vi "Stanford Research SR1 Quick Measurements.vi"() -> ()   [LabVIEW 2014]
doc: "This example shows how to configure a Quick Measurement for a free-run and set up a basic structure for stopping and resuming the Distortion Quick Measurement."
uses:
  Stanford Research SR1.lvlib
panel:
  in  "Pause / Resume":bool
  in  "Stop":bool
  in  "Number Of Steps (0)":i32
  in  "Stop Frequency (10 Hz)":dbl=10.0
  in  "Start Frequency (10 Hz)":dbl=10.0
  in  "Waveform (0: wsSine)":i32(ring) items=["wsSine", "wsLDSine"]
  in  "VISA resource name":refnum<visa-resource-name>
  # "(c) 2014 National Instruments.  ALL RIGHTS RESERVED."
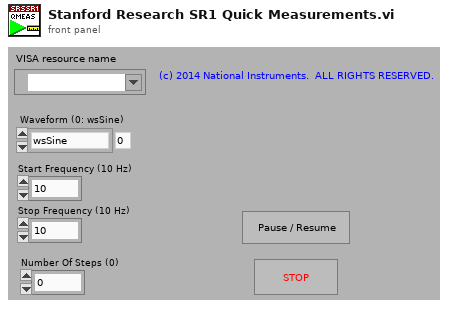
[diagram p1: front panel]
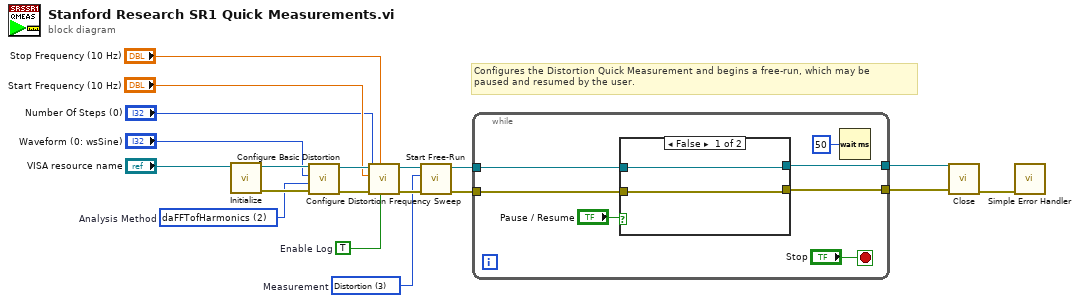
[diagram p0: block diagram]
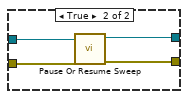
[diagram p2: hidden frame]
diagram:
  w6 = 2 items=["daTHD", "daHarmonics", "daFFTofHarmonics"]  # Analysis Method
  w7 = TRUE  # Enable Log
  w8 = 3 items=["Level", "SNR", "THDN", "Distortion", "IMDistortion", "Crosstalk", "FrequencyResponse", "InputOutputPhase", "InterchannelPhase"]  # Measurement
  # "Configures the Distortion Quick Measurement and begins a free-run, which may be \npaused and resumed by the user."
  n1 = call "Initialize.vi"("VISA resource name"="VISA resource name") -> ("error out"=w16:errorcluster, "VISA resource name out"=w17:refnum<visa-resource-name>)  [unwired: 9 in]
  n2 = call "Configure Basic Distortion.vi"("error in (no error)"=w16, "Analysis Method (0: daTHD)"=w6, "Waveform (0: wsSine)"="Waveform (0: wsSine)", "VISA resource name"=w17) -> ("error out"=w13:errorcluster, "VISA resource name out"=w14:refnum<visa-resource-name>)  [unwired: 6 in]
  n3 = call "Configure Distortion Frequency Sweep.vi"("Enable Log (F: Disabled)"=w7, "Stop Frequency (10 Hz)"="Stop Frequency (10 Hz)", "error in (no error)"=w13, "Number Of Steps (0)"="Number Of Steps (0)", "Start Frequency (10 Hz)"="Start Frequency (10 Hz)", "VISA resource name"=w14) -> ("error out"=w9:errorcluster, "VISA resource name out"=w10:refnum<visa-resource-name>)  [unwired: 4 in]
  n4 = call "Start Free-Run.vi"("error in (no error)"=w9, "Measurement (0: Level)"=w8, "VISA resource name"=w10) -> ("error out"=w3:errorcluster, "VISA resource name out"=w4:refnum<visa-resource-name>)  [unwired: 7 in]
  n5 = while {
    tunnel: w4 -> [w24]
    tunnel: w3 -> [w23]
    tunnel: [w22] -> w2
    tunnel: [w21] -> w1
    stop <- "Stop" stop-if-true
    n6 = case shown="False" "Pause / Resume" {
      tunnel: w24 -> [w28 w32]
      tunnel: w23 -> [w27 w31]
      tunnel: [w28 w30] -> w22
      tunnel: [w27 w29] -> w21
      frame False {
      }
      frame True {
        n7 = call "Pause Or Resume Sweep.vi"("error in (no error)"=w31, "VISA resource name"=w32) -> ("error out"=w29:errorcluster, "VISA resource name out"=w30:refnum<visa-resource-name>)  [unwired: 8 in]
      }
    }
    n8 = Wait (ms)(milliseconds to wait=u32 50) -> ()  [unwired: 1 out]
  }
  n9 = call "Close.vi"("error in (no error)"=w1, "VISA resource name"=w2) -> ("error out"=w18:errorcluster)  [unwired: 9 in]
  n10 = call <vilib>:"Simple Error Handler.vi"("error in (no error)"=w18) -> ()  [unwired: 4 in, 5 out]
